vi "Configure Modulation (Frequency Shift-Keying).vi"(0 "VISA resource name":refnum<visa-resource-name>, 1 "Enable Frequency Shift-keying Modulation (T:Enable)":bool, 5 "Channel (1: Channel1)":u16(ring) items=["Channel1", "Channel2"], 7 "FSKM Source (0: Internal)":u16(ring) items=["Internal", "Other Channel", "External"], 9 "Internal Rate (1000.0 Hz)":dbl, 11 "error in (no error)":errorcluster, 12 "Hop Frequency (1000.0 Hz)":dbl) -> (4 "VISA resource name out":refnum<visa-resource-name>, 15 "error out":errorcluster)   [LabVIEW 2009, in "Agilent 81150.lvlib"]
doc: "Configures and enables Frequency-Shift Keying (FSK) modulation. The function generator shifts its output frequency between two present values.\n\n<B>Note(s):</B>\nThe Pulse, Noise, and DC waveform functions are not valid for Configure Modulation (Frequency Shift Keying)."
uses:
  Agilent 81150.lvlib
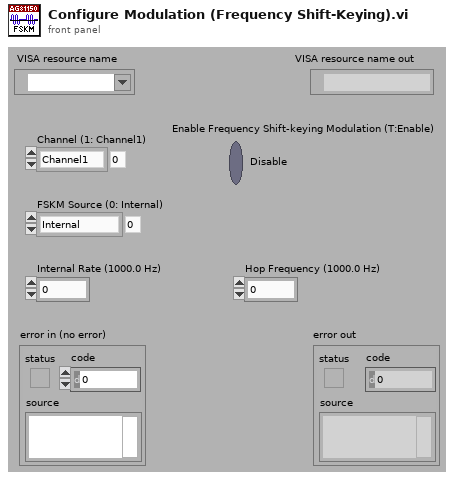
[diagram p1: front panel]
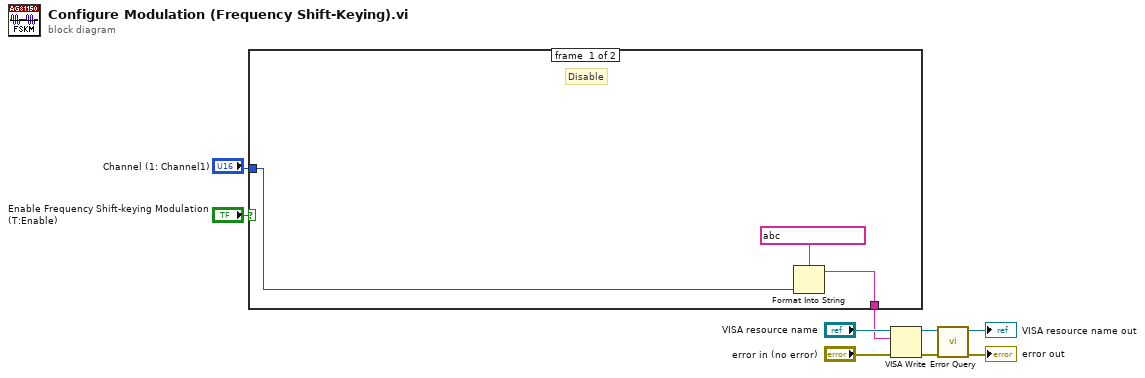
[diagram p0: block diagram]
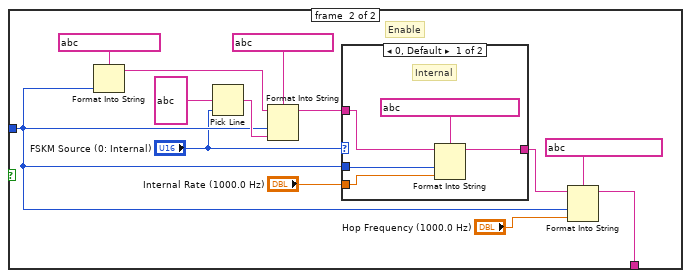
[diagram p2: hidden frame]
diagram:
  n1 = case shown="True" "Enable Frequency Shift-keying Modulation (T:Enable)" {
    tunnel: [w10 w14] -> w3
    tunnel: "Channel (1: Channel1)" -> [w11 w18]
    frame #0 {
      # "Disable"
      n2 = Format Into String(format string=string ?, w11) -> (resulting string=w10:string)  [unwired: 2 in, 1 out]
    }
    frame #1 {
      # "Enable"
      n3 = Format Into String(format string=string ?, w18) -> (resulting string=w13:string)  [unwired: 2 in, 1 out]
      n4 = Pick Line(multi-line string=string ?, line index="FSKM Source (0: Internal)") -> (output string=w19:string)  [unwired: 1 out]
      n5 = Format Into String(format string=string ?, initial string=w13, w18, w19) -> (resulting string=w21:string)  [unwired: 1 in, 1 out]
      n6 = case shown="0, Default" "FSKM Source (0: Internal)" {
        tunnel: w18 -> [w28 _]
        tunnel: [w29 w31] -> w24
        tunnel: w21 -> [w27 w31]
        tunnel: "Internal Rate (1000.0 Hz)" -> [w26 _]
        frame #0 {
          # "Internal"
          n7 = Format Into String(format string=string ?, initial string=w27, w28, w26) -> (resulting string=w29:string)  [unwired: 1 in, 1 out]
        }
        frame #1 {
          # "Other Channel or External"
        }
      }
      n8 = Format Into String(format string=string ?, initial string=w24, w18, "Hop Frequency (1000.0 Hz)") -> (resulting string=w14:string)  [unwired: 1 in, 1 out]
    }
  }
  n9 = VISA Write(VISA resource name="VISA resource name", write buffer=w3, error in (no error)="error in (no error)") -> (VISA resource name out=w5:refnum<visa-resource-name>, error out=w4:errorcluster)  [unwired: 1 out]
  n10 = call "Error Query.vi"("error in (no error)"=w4, "VISA resource name"=w5) -> ("error out"=→"error out":errorcluster, "VISA resource name out"=→"VISA resource name out":refnum<visa-resource-name>)  [unwired: 8 out]
